vi "Harmonics MSMT Configure Relative Power Step.vi"(8 "error in (no error)":errorcluster, 10 "Export Data Locations":string[](array[string]), 11 "Harmonics in":refnum<class "Harmonics.lvclass">) -> (0 "error out":errorcluster, 3 "Harmonics out":refnum<class "Harmonics.lvclass">)   [LabVIEW 2018, in "Harmonics.lvlib" / "Harmonics.lvclass"]
uses:
  Harmonics.lvclass
  C:/Sequence Automation/Plugins/Measurement Interface.lvlibp/Measurement Interface.lvclass
  Harmonics.lvclass/Harmonics.ctl
  Protected Methods/Read Harmonics.vi
  Plugins/Measurement Interface.lvlibp/Private Methods/Engine Reference/Read Engine Reference.vi
  Plugins/Measurement Interface.lvlibp/Private Methods/Measurement Name/Read Measurement Name.vi
  Plugins/Measurement Interface.lvlibp/Private Methods/Measurement Parameters/Read Measurement Parameters.vi
  Plugins/String Database.lvlibp/String Database.lvclass
  Evaluations/Harmonics/Harmonics_Relative_Power/Harmonics_Relative_Power.lvclass
  Plugins/TestStand API Tools (TSAT).lvlibp/Step Actions/TSAT Step Actions.lvlib
  Plugins/Test Number and Bin Generator.lvlibp/Test Number and Bin Generator/Test Number and Bin Generator.lvclass
  Plugins/Measurement Interface.lvlibp/Measurement Interface.lvclass
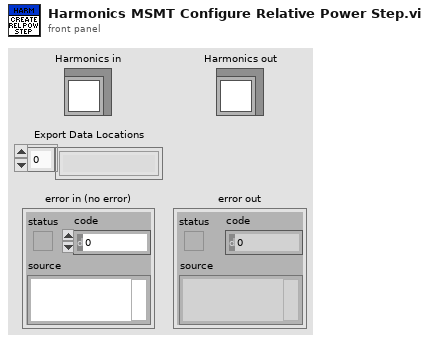
[diagram p1: front panel]
types:
  T1 = typedef "TestStand API Tools (TSAT).lvlibp/TSAT Evaluation Actions.lvlib/TSAT Evaluation.ctl" = cluster{"Test Name":string, "Pin":string, "Units":string, "SI Scaling":T2, "Test Number":i32, "Published Data Id":string, "Low Limit":dbl, "High Limit":dbl, "Export Data Location":string, "Software Bin":i64, "Evaluation Type":T3, "Test Data Source":string}
  T2 = typedef "TestStand API Tools (TSAT).lvlibp/TSAT Evaluation Actions.lvlib/TSAT Eval SI Unit Scaling.ctl" = i16
  T3 = typedef "TestStand API Tools (TSAT).lvlibp/TSAT Evaluation Actions.lvlib/TSAT Evaluation Type.ctl" = enum16{"Numeric Limit", "Pass/Fail", "None"}
  T4 = typedef "Test Number and Bin Generator.lvlibp/Test Number and Bin Generator.lvclass/Session Handle.ctl" = refnum<data-value>
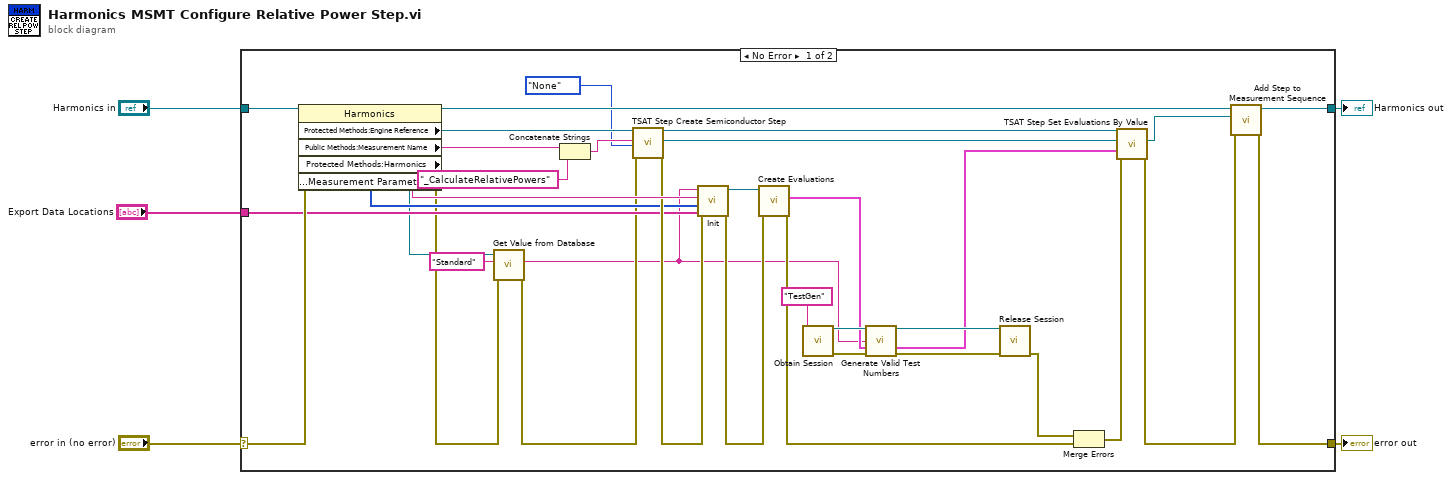
[diagram p0: block diagram]
diagram:
  n1 = case shown="No Error" "error in (no error)" {
    selector: "error in (no error)" -> [w39 w41]
    tunnel: [w34 w41] -> w4
    tunnel: [w32 w40] -> w2
    tunnel: "Harmonics in" -> [w38 w40]
    tunnel: "Export Data Locations" -> [w28 _]
    frame No Error {
      n2 = property class="Harmonics"(reference=w38, error in=w39) -> (reference out=w33:refnum<class "Harmonics.lvclass">, error out=w14:errorcluster, "Protected Methods:Engine Reference"=w37:refnum<k7>, "Public Methods:Measurement Name"=w31:string, "Protected Methods:Harmonics"=w29:i8[], "Protected Methods:Measurement Parameters"=w15:refnum<class "String Database.lvclass">)
      n3 = call "Get Value from Database.vi"("error in (no error)"=w14, "Entry Name"="Standard", "Message in"=w15) -> ("error out"=w13:errorcluster, "Entry Value"=w7:string)  [unwired: 5 in, 2 out]
      n4 = Concatenate Strings(w31, "_CalculateRelativePowers" ("string")) -> (w35:string)
      n5 = call "TSAT Step Create Semiconductor Step.vi"("Engine In"=w37, "Step Name"=w35, "Module Type"=enum16{"None", "DotNet", "LabVIEW"}."None", "Error In"=w13) -> ("Engine Out"=w21:refnum<k7>, "Step Reference"=w23:refnum<k7>, "Error Out"=w30:errorcluster)  [unwired: 13 in]
      n6 = call "Init.vi"("Export Data Locations"=w28, "error in (no error)"=w30, "Harmonics"=w29, "Measurement Name"=w31, "Standard"=w7) -> ("error out"=w27:errorcluster, "Harmonics_Relative_Power out"=w26:refnum<class "Harmonics_Relative_Power.lvclass">)  [unwired: 5 in]
      n7 = call-dynamic "Create Evaluations.vi"("error in (no error)"=w27, "IEvaluation in"=w26) -> ("error out"=w25:errorcluster, "Evaluations Out"=w11:T1[])  [unwired: 7 in, 1 out]
      n8 = call "Obtain Session.vi"("Session  Name ()"="TestGen") -> ("Session Handle"=w19:T4, "error out"=w16:errorcluster)  [unwired: 13 in]
      n9 = call "Generate Valid Test Numbers.vi"("Session Handle in"=w19, "Test Group"=w7, "Evaluations In"=w11, "error in (no error)"=w16) -> ("Session Handle out"=w18:T4, "Evaluations Out"=w10:T1[], "error out"=w17:errorcluster)  [unwired: 9 in]
      n10 = call "Release Session.vi"("Session Handle"=w18, "error in (no error)"=w17) -> ("error out"=w8:errorcluster)  [unwired: 13 in]
      n11 = Merge Errors(w8, w25) -> (w9:errorcluster)
      n12 = call "TSAT Step Set Evaluations By Value.vi"("Error In"=w9, "Evaluation Data"=w10, "Step In"=w23, "Engine In"=w21) -> ("Error Out"=w24:errorcluster, "Step Out"=w22:refnum<k7>)  [unwired: 5 in, 1 out]
      n13 = call "Add Step to Measurement Sequence.vi"("error in (no error)"=w24, "Step to Add"=w22, "Measurement Interface in"=w33) -> ("error out"=w34:errorcluster, "Measurement Interface out"=w32:refnum<class "Harmonics.lvclass">)  [unwired: 7 in]
    }
    frame Error {
    }
  }
  "error out" <- w4
  "Harmonics out" <- w2
